vi "Check Conflict Zones.vi"(8 "error in (no error)":errorcluster, 11 "VacuumLines in":refnum<class "VacuumLines.lvclass">) -> (0 "error out":errorcluster, 3 "VacuumLines out":refnum<class "VacuumLines.lvclass">)   [LabVIEW 2016, in "Hardware.lvlib" / "VacuumLine.lvlib" / "VacuumLines.lvclass"]
uses:
  <userlib>/Common Components/Hardware/Abstract System/VacuumLine/VacuumLines/VacuumLines.lvclass
  <userlib>/Common Components/Hardware/Abstract System/VacuumLine/VacuumLines/VacuumLines.lvclass/VacuumLines.ctl
  <userlib>/Common Components/Hardware/Abstract System/VacuumLine/VacuumLine/VacuumLine.lvclass/VacuumLine.ctl
  <userlib>/Common Components/Hardware/Abstract System/VacuumLine/VacuumLine/Read Current DispSnsr Value.vi
  <userlib>/Common Components/Hardware/Abstract System/VacuumLine/VacuumLine/Read Soft Moving Status.vi
  <userlib>/Common Components/Hardware/Abstract System/VacuumLine/VacuumLine/VacuumLine.lvclass
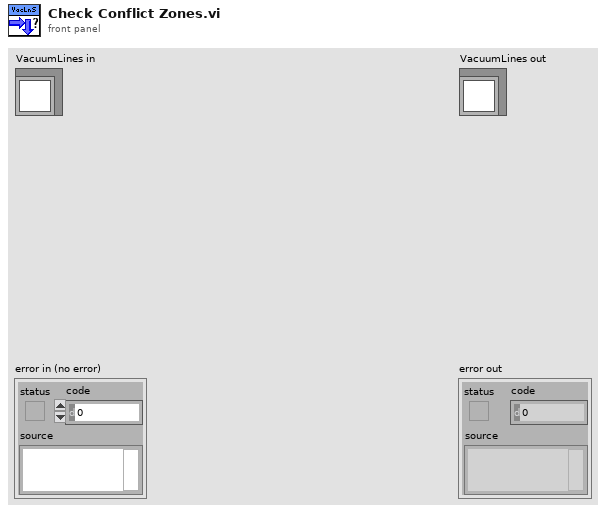
[diagram p1: front panel]
types:
  T1 = typedef "Hardware.lvlib/VacuumLine.lvlib/VacuumLines.lvclass/Conflict Zone.ctl" = cluster{"1":cluster{"Label":string, "from":dbl, "to":dbl, "buffer":dbl}, "2":cluster{"Label":string, "from":dbl, "to":dbl, "buffer":dbl}}
  T2 = cluster{"Label":string, "from":dbl, "to":dbl, "buffer":dbl}[]
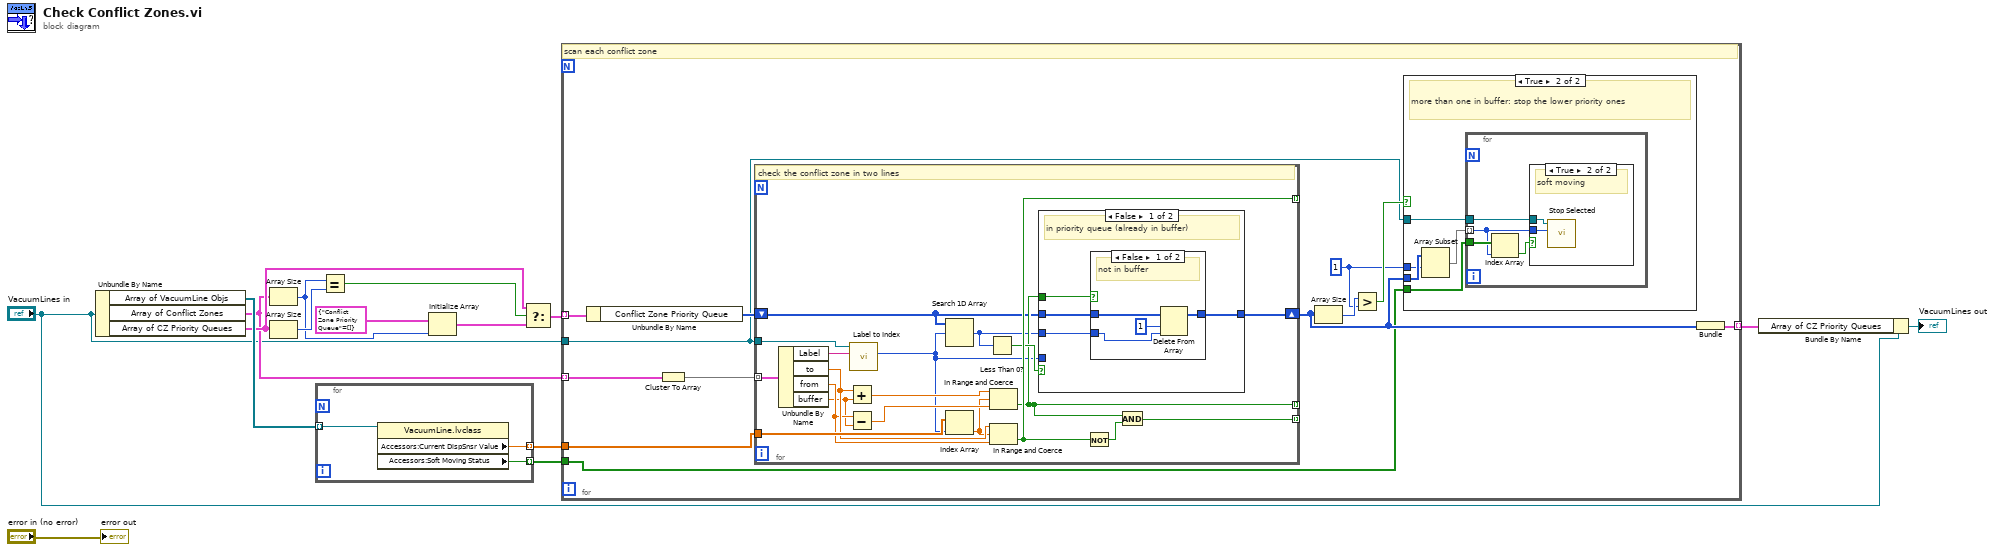
[diagram p0: block diagram]
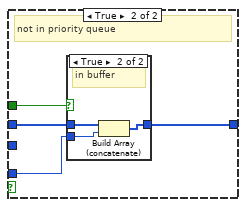
[diagram p5: hidden frame]
diagram:
  n1 = Unbundle By Name("VacuumLines in") -> ("Array of VacuumLine Objs"=w13:refnum<class "VacuumLine.lvclass">[], "Array of Conflict Zones"=w6:T1[], "Array of CZ Priority Queues"=w10:cluster{"Conflict Zone Priority Queue":i32[]}[])
  n2 = Array Size(array=w6) -> (size(s)=w9:i32)
  n3 = Array Size(array=w10) -> (size(s)=w12:i32)
  n4 = for {
    tunnel: w13 -> [w18] mode=indexing
    tunnel: [w17] -> w3 mode=indexing
    tunnel: [w16] -> w1 mode=indexing
    n5 = property class="VacuumLine.lvclass"(reference=w18) -> ("Accessors:Current DispSnsr Value"=w17:dbl, "Accessors:Soft Moving Status"=w16:bool)  [unwired: 1 in, 2 out]
  }
  n6 = Equal?(x=w9, y=w12) -> (x = y?=w11:bool)
  n7 = Initialize Array(cluster{"Conflict Zone Priority Queue":i32[]} {"Conflict Zone Priority Queue"=[]} ("Cluster"), w9) -> (w7:cluster{"Conflict Zone Priority Queue":i32[]}[])
  n8 = Select(t=w10, s=w11, f=w7) -> (s? t:f=w5:cluster{"Conflict Zone Priority Queue":i32[]}[])
  n9 = for {
    tunnel: w6 -> [w30] mode=indexing
    tunnel: w5 -> [w27] mode=indexing
    tunnel: "VacuumLines in" -> [w20]
    tunnel: w3 -> [w28]
    tunnel: [w25] -> w2 mode=indexing
    tunnel: w1 -> [w19]
    w21 = 1 ("y")
    # "scan each conflict zone"
    n10 = Unbundle By Name(w27) -> ("Conflict Zone Priority Queue"=w26:i32[])
    n11 = Cluster To Array(cluster=w30) -> (array=w29:T2)
    n12 = for {
      tunnel: w29 -> [w51] mode=indexing
      tunnel: w20 -> [w60]
      tunnel: w28 -> [w59]
      tunnel: [w49] -> _ mode=indexing
      tunnel: [w48] -> _ mode=indexing
      shift-right: [w42] -> w22
      shift-left: w26 -> [w45]
      tunnel: [w46] -> _ mode=indexing
      # "check the conflict zone in two lines"
      n13 = Unbundle By Name(w51) -> ("Label"=w50:string, "to"=w58:dbl, "from"=w56:dbl, "buffer"=w55:dbl)
      n14 = Add(x=w58, y=w55) -> (x+y=w57:dbl)
      n15 = Subtract(x=w56, y=w55) -> (x-y=w54:dbl)
      n16 = call <userlib>:"Label to Index.vi"("Label"=w50, "VacuumLines in"=w60) -> ("Index"=w44:i32)  [unwired: 7 in, 2 out]
      n17 = Search 1D Array(1D array=w45, element=w44) -> (index of element=w43:i32)  [unwired: 1 in]
      n18 = Index Array(array=w59, index=w44) -> (element=w52:dbl)
      n19 = Less Than 0?(x=w43) -> (x < 0?=w47:bool)
      n20 = In Range and Coerce(upper limit=w57, x=w52, lower limit=w54) -> (In Range?=w46:bool)  [unwired: 1 out]
      n21 = In Range and Coerce(upper limit=w58, x=w52, lower limit=w56) -> (In Range?=w49:bool)  [unwired: 1 out]
      n22 = case shown="False" w47 {
        tunnel: w46 -> [w64 w73]
        tunnel: w45 -> [w63 w72]
        tunnel: w44 -> [_ w71]
        tunnel: [w62 w70] -> w42
        tunnel: w43 -> [w61 _]
        frame False {
          # "in priority queue (already in buffer)"
          n23 = case shown="False" w64 {
            tunnel: w63 -> [w68 w69]
            tunnel: [w65 w69] -> w62
            tunnel: w61 -> [w67 _]
            frame False {
              # "not in buffer"
              n24 = Delete From Array(array=w68, length=1, index=w67) -> (array with subset deleted=w65:i32[])  [unwired: 1 out]
            }
            frame True {
              # "in buffer"
            }
          }
        }
        frame True {
          # "not in priority queue"
          n25 = case shown="True" w73 {
            tunnel: w72 -> [w74 w77]
            tunnel: w71 -> [_ w76]
            tunnel: [w74 w75] -> w70
            frame False {
              # "not in buffer"
            }
            frame True {
              # "in buffer"
              n26 = Build Array (concatenate)(w77, w76) -> (w75:i32[])
            }
          }
        }
      }
      n27 = Not(x=w49) -> (.not. x?=w53:bool)
      n28 = And(x=w46, y=w53) -> (x .and. y?=w48:bool)
    }
    n29 = Array Size(array=w22) -> (size(s)=w24:i32)
    n30 = Greater?(x=w24, y=w21) -> (0:w23:bool)
    n31 = case shown="True" w23 {
      tunnel: w22 -> [_ w35]
      tunnel: w21 -> [_ w34]
      tunnel: w20 -> [_ w32]
      tunnel: w19 -> [_ w31]
      frame False {
      }
      frame True {
        # "more than one in buffer: stop the lower priority ones"
        n32 = Array Subset(array=w35, index=w34) -> (w33:i32[])  [unwired: 1 in]
        n33 = for {
          tunnel: w33 -> [w37] mode=indexing
          tunnel: w32 -> [w39]
          tunnel: w31 -> [w38]
          n34 = Index Array(array=w38, index=w37) -> (element=w36:bool)
          n35 = case shown="True" w36 {
            tunnel: w39 -> [_ w41]
            tunnel: w37 -> [_ w40]
            frame False {
            }
            frame True {
              # "soft moving"
              n36 = call <userlib>:"Stop Selected.vi"("index"=w40, "VacuumLines in"=w41) -> ()  [unwired: 8 in, 2 out]
            }
          }
        }
      }
    }
    n37 = Bundle("Conflict Zone Priority Queue"=w22) -> (w25:cluster{"Conflict Zone Priority Queue":i32[]})  [unwired: 1 in]
  }
  n38 = Bundle By Name(cluster="VacuumLines in", "Array of CZ Priority Queues"=w2) -> (→"VacuumLines out":refnum<class "VacuumLines.lvclass">)
  "error out" <- "error in (no error)"
